vi "Get Boolean.vi"(8 "error in (no error)":errorcluster, 11 "BooleanMsg in":refnum<class "BooleanMsg.lvclass">) -> (0 "error out":errorcluster, 2 "Message Data":bool, 3 "BooleanMsg out":refnum<class "BooleanMsg.lvclass">)   [LabVIEW 2017, in "LapDog.Messaging.v3.NativeTypes.lvlib" / "BooleanMsg.lvclass"]
doc: "Returns the data contained in the message.\n\nThis method executes regardless of the error in state."
uses:
  BooleanMsg.lvclass
  BooleanMsg.lvclass/BooleanMsg.ctl
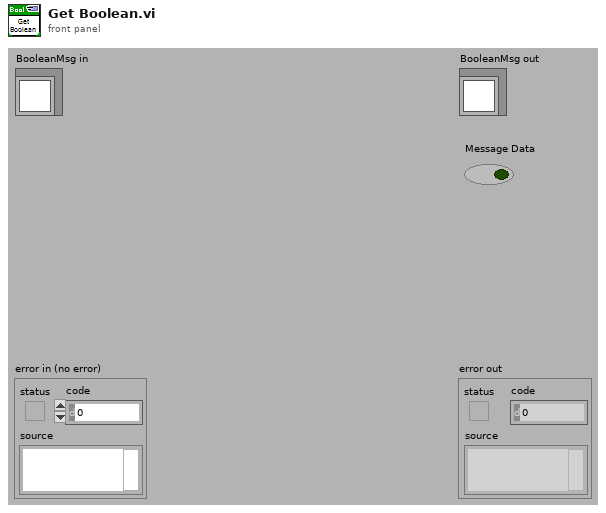
[diagram p1: front panel]
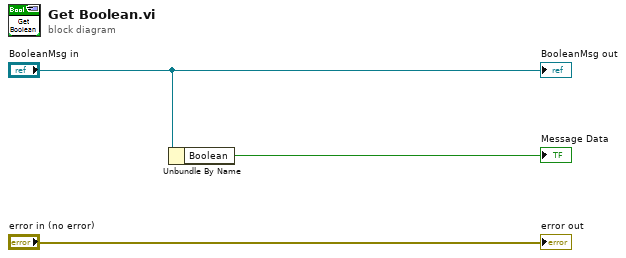
[diagram p0: block diagram]
diagram:
  n1 = Unbundle By Name("BooleanMsg in") -> ("Boolean"=→"Message Data":bool)
  "error out" <- "error in (no error)"
  "BooleanMsg out" <- "BooleanMsg in"
